vi "연속읽기(Main).vi"() -> ()   [LabVIEW 2014]
panel:
  out "Word 배열":u16[](array[numeric]) format="%.0x"
  out "에러 출력":errorcluster
  in  "데이터개수(Byte)":u16=50
  in  "직접변수(Byte)":string="%DB0000"
  in  "주소":string="192.168.0.10"
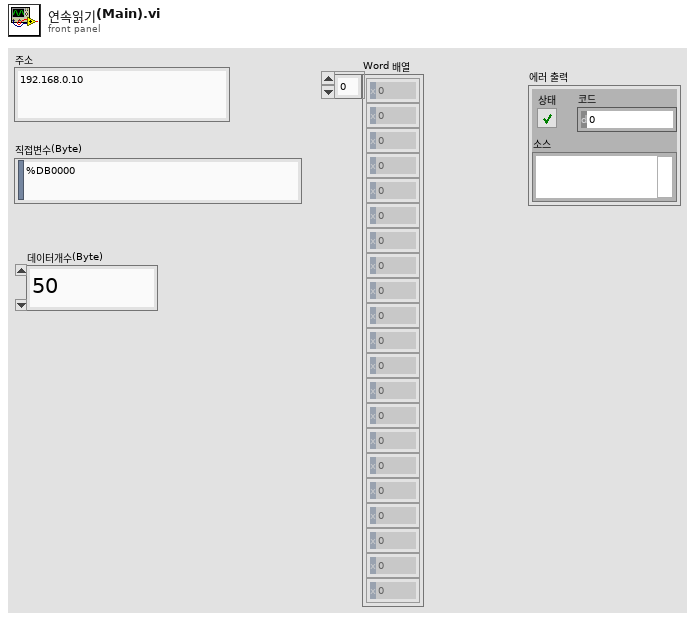
[diagram p1: front panel]
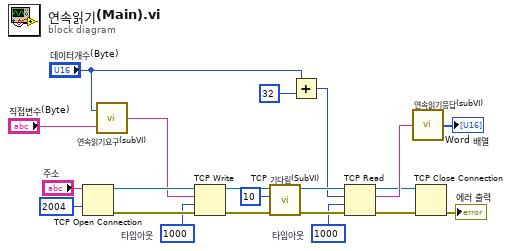
[diagram p0: block diagram]
diagram:
  w1 = 1000  # 타임아웃
  w5 = 1000  # 타임아웃
  n1 = TCP Open Connection(address="주소", remote port or service name=u16 2004 ("원격 포트 또는 서비스 이름")) -> (connection ID=w19:refnum<k5>, error out=w18:errorcluster)  [unwired: 3 in]
  n2 = call "연속읽기요구(subVI).vi"("직접변수(Byte)"="직접변수(Byte)", "데이터개수(Byte)"="데이터개수(Byte)") -> ("연속읽기"=w17:string)
  n3 = TCP Write(connection ID=w19, data in=w17, error in (no error)=w18, 9:w5) -> (connection ID out=w14:refnum<k5>, error out=w13:errorcluster)  [unwired: 1 out]
  n4 = call "TCP 기다림(SubVI).vi"("error in"=w13, "기다림(ms)"=u32 10, "TCP 네트워크 연결 입력"=w14) -> ("error out"=w10:errorcluster, "TCP 네트워크 연결 출력"=w11:refnum<k5>)  [unwired: 7 in]
  n5 = Add(x="데이터개수(Byte)", y=u16 32 ("x")) -> (x+y=w3:u16)
  n6 = TCP Read(connection ID=w11, bytes to read=w3, error in (no error)=w10, 9:w1) -> (connection ID out=w8:refnum<k5>, data out=w9:string, error out=w7:errorcluster)  [unwired: 1 in]
  n7 = call "연속읽기응답(subVI).vi"("응답프레임"=w9) -> ("Word 배열"=→"Word 배열":u16[])
  n8 = TCP Close Connection(connection ID=w8, error in (no error)=w7) -> (error out=→"에러 출력":errorcluster)  [unwired: 1 in, 1 out]
